vi "Stopwatch.vi"(0 "Start":bool, 5 "Resume":bool, 7 "Pause":bool, 9 "Reset":bool, 11 "Stop":bool) -> (4 "hour":dbl, 6 "min":dbl, 8 "sec":u8, 10 "ms":dbl)   [LabVIEW 2020]
panel:
  # "Description:\n1. Use Start to start the stopwatch. \n2. You can pause and resume the stopwatch using stop and reusm button.\n3. Use Stop to stop the stopwatch."
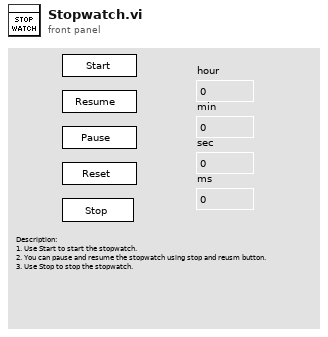
[diagram p1: front panel]
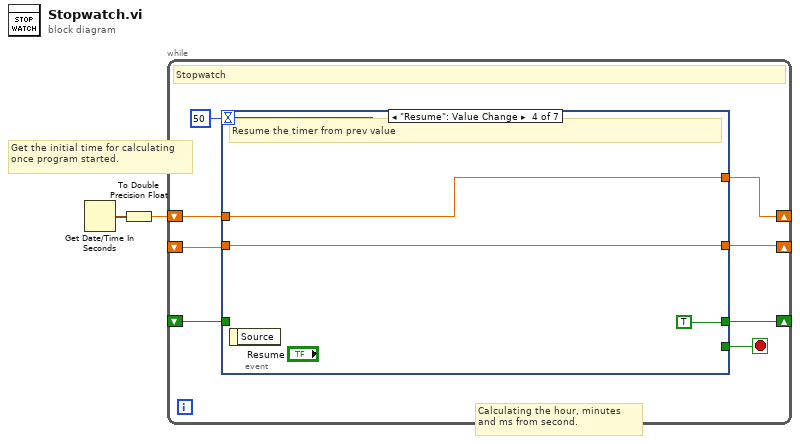
[diagram p0: block diagram]
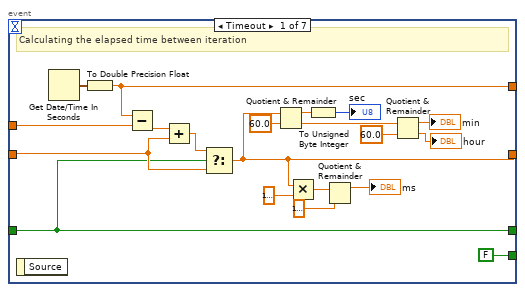
[diagram p2: hidden frame]
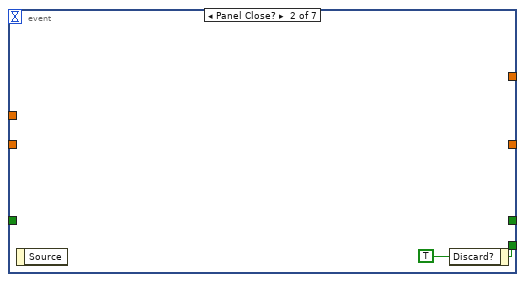
[diagram p3: hidden frame]
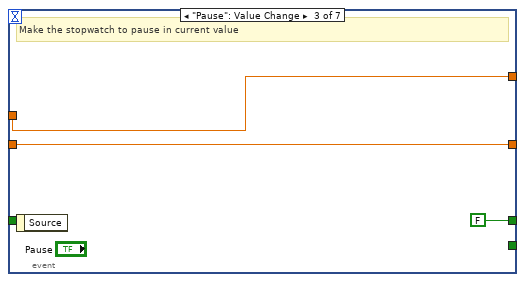
[diagram p4: hidden frame]
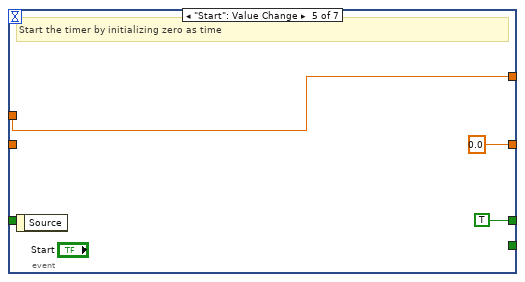
[diagram p5: hidden frame]
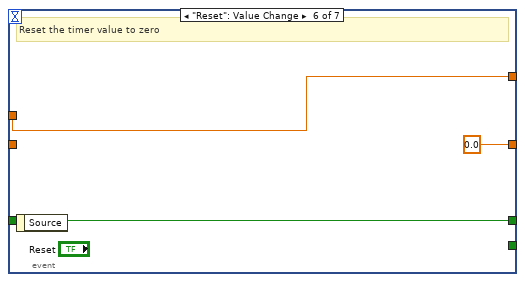
[diagram p6: hidden frame]
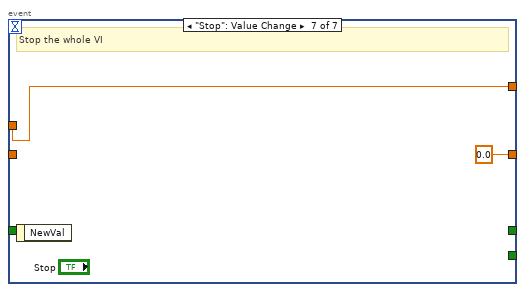
[diagram p7: hidden frame]
diagram:
  # "Calculating the hour, minutes and ms from second."
  # "Get the initial time for calculating once program started."
  n1 = Get Date/Time In Seconds() -> (seconds since 1Jan1904=w2:timestamp)
  n2 = To Double Precision Float(number=w2) -> (double precision float=w1:dbl)
  n3 = while {
    shift-right: [w3] -> _
    shift-left: _ -> [w8]
    shift-right: [w6] -> _
    shift-left: w1 -> [w7]
    shift-right: [w4] -> _
    shift-left: _ -> [w5]
    stop <- w9 stop-if-true
    # "Stopwatch"
    n4 = event shown="[3] \"Resume\": Value Change" {
      selector: _ -> [_ _ _ _ _ _ _]
      dyn-events: _ -> [_ _ _ _ _ _ _]
      timeout: 50 -> [_ _ _ _ _ _ _]
      tunnel: [FALSE w31 _ _ _ _ _] -> w9
      tunnel: w8 -> [w24 _ w33 w36 _ _ _]
      tunnel: w7 -> [w27 _ w34 w37 w38 w42 w44]
      tunnel: [w26 _ w34 w37 w38 w42 w44] -> w6
      tunnel: [w14 _ w33 w36 0.0 0.0 0.0] -> w3
      tunnel: w5 -> [w23 _ _ _ _ w41 _]
      tunnel: [w23 _ FALSE TRUE TRUE w41 _] -> w4
      event Timeout {
        # "Calculating the elapsed time between iteration"
        n5 = event-data() -> ()  [unwired: 1 in, 1 out]
        n6 = Get Date/Time In Seconds() -> (seconds since 1Jan1904=w29:timestamp)
        n7 = To Double Precision Float(number=w29) -> (double precision float=w26:dbl)
        n8 = Subtract(x=w26, y=w27) -> (x-y=w28:dbl)
        n9 = Add(x=w28, y=w24) -> (x+y=w25:dbl)
        n10 = Select(t=w25, s=w23, f=w24) -> (s? t:f=w14:dbl)
        n11 = Quotient & Remainder(x=w14, y=60.0) -> (x-y*floor(x/y)=w16:dbl, floor(x/y)=w21:dbl)
        n12 = Multiply(x=w14, y=1000.0) -> (x*y=w22:dbl)
        n13 = To Unsigned Byte Integer(number=w16) -> (unsigned 8bit integer=→"sec":u8)
        n14 = Quotient & Remainder(x=w22, y=1000.0) -> (x-y*floor(x/y)=→"ms":dbl)  [unwired: 1 out]
        n15 = Quotient & Remainder(x=w21, y=60.0) -> (x-y*floor(x/y)=→"min":dbl, floor(x/y)=→"hour":dbl)
      }
      event Panel Close? {
        w31 = TRUE ("Discard?")
        n16 = event-data() -> ()  [unwired: 1 in, 1 out]
        n17 = event-data("Discard?"=w31) -> ()  [unwired: 1 in, 1 out]
      }
      event "Pause": Value Change {
        # "Make the stopwatch to pause in current value"
        n18 = event-data() -> ()  [unwired: 1 in, 1 out]
      }
      event "Resume": Value Change {
        # "Resume the timer from prev value"
        n19 = event-data() -> ()  [unwired: 1 in, 1 out]
      }
      event "Start": Value Change {
        # "Start the timer by initializing zero as time"
        n20 = event-data() -> ()  [unwired: 1 in, 1 out]
      }
      event "Reset": Value Change {
        # "Reset the timer value to zero"
        n21 = event-data() -> ()  [unwired: 1 in, 1 out]
      }
      event "Stop": Value Change {
        # "Stop the whole VI"
        n22 = event-data() -> ()  [unwired: 1 in, 1 out]
      }
    }
  }
